vi "SwerveDriveLogic.vi"(8 "Joystick Axes":dbl[](array[numeric]), 9 "Speeds":dbl[](array[numeric]), 10 "AngleSetpoints":dbl[](array[numeric]), 11 "AngleEncoders":dbl[](array[numeric])) -> (2 "AngleMotorsReversed":bool[](array[boolean]), 3 "AngleMotorOutputs":dbl[](array[numeric]))   [LabVIEW 2018]
uses:
  <vilib>/addons/control/pid/pid.llb/PID (DBL).vi
  <vilib>/addons/control/pid/NI_PID_pid.lvlib
panel:
  out "Back right module":dbl(knob)
  out "Back left module":dbl(knob)
  out "Front left module":dbl(knob)
  out "Front right module":dbl(knob)
  in  "PID gains":T1={"proportional gain (Kc)"=0.02, "integral time (Ti, min)"=0.0, "derivative time (Td, min)"=0.0} {"derivative time (Td, min)" format="%.15f"; "integral time (Ti, min)" format="%.3f"; "proportional gain (Kc)" format="%.3f"}
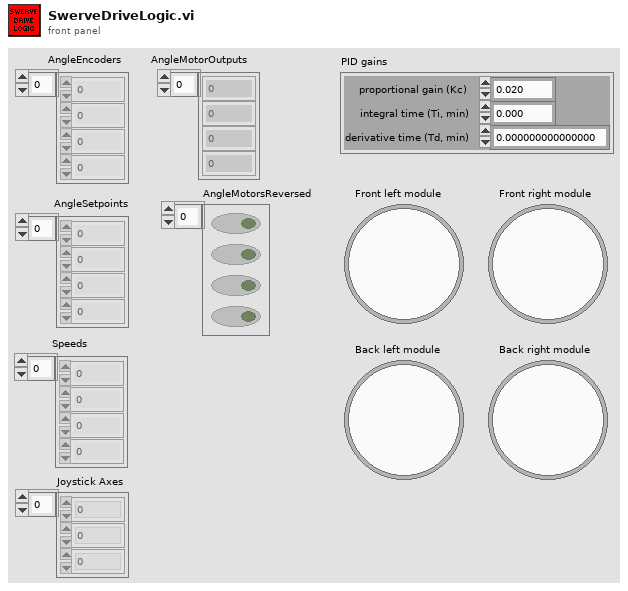
[diagram p1: front panel]
types:
  T1 = cluster{"proportional gain (Kc)":dbl, "integral time (Ti, min)":dbl, "derivative time (Td, min)":dbl}
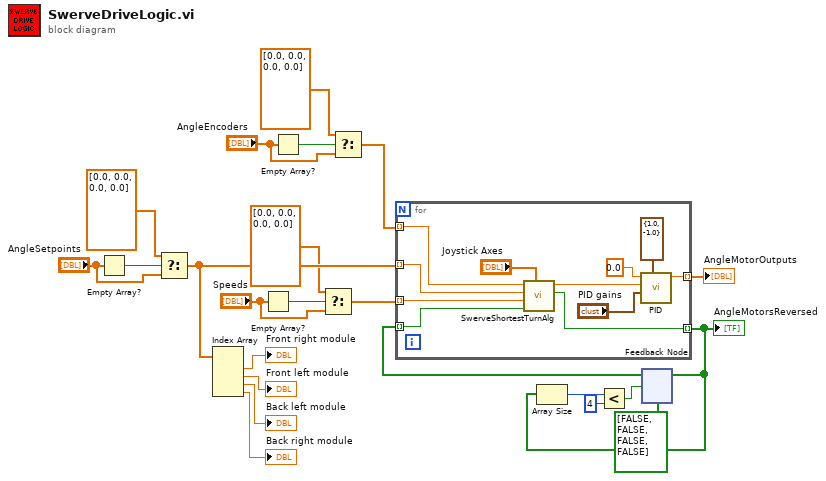
[diagram p0: block diagram]
diagram:
  n1 = Empty Array?(array="AngleSetpoints") -> (empty?=w15:bool)
  n2 = Select(t=dbl[] [0.0, 0.0, 0.0, 0.0] ("AngleSetpoints"), s=w15, f="AngleSetpoints") -> (s? t:f=w14:dbl[])
  n3 = Index Array(array=w14) -> (element #1=→"Front right module":dbl, element #2=→"Front left module":dbl, element #3=→"Back left module":dbl, element #4=→"Back right module":dbl)  [unwired: 4 in]
  n4 = Empty Array?(array="Speeds") -> (empty?=w12:bool)
  n5 = Empty Array?(array="AngleEncoders") -> (empty?=w18:bool)
  n6 = Select(t=dbl[] [0.0, 0.0, 0.0, 0.0] ("AngleSetpoints"), s=w12, f="Speeds") -> (s? t:f=w10:dbl[])
  n7 = Select(t=dbl[] [0.0, 0.0, 0.0, 0.0] ("AngleSetpoints"), s=w18, f="AngleEncoders") -> (s? t:f=w7:dbl[])
  n8 = feedback #1(bool[] [FALSE, FALSE, FALSE, FALSE]) -> (w3:bool[])
  n9 = for {
    tunnel: w3 -> [w29] mode=indexing
    tunnel: w14 -> [w31] mode=indexing
    tunnel: [w33] -> w23 mode=indexing
    tunnel: [w25] -> w2 mode=indexing
    tunnel: w7 -> [w28] mode=indexing
    tunnel: w10 -> [w27] mode=indexing
    n10 = call "SwerveShortestTurnAlg.vi"("Joystick Axes"="Joystick Axes", "SwerveMotorsFlipped?"=w29, "SwerveSpeed"=w27, "AngleSetpoint"=w31, "AngleEncoder"=w28) -> ("FlipSwerveMotors"=w25:bool, "PIDInput"=w26:dbl)  [unwired: 5 in]
    n11 = call-poly <vilib>:"PID.vi"("output range"=cluster{"output high":dbl, "output low":dbl} {"output high"=1.0, "output low"=-1.0}, "PID gains"="PID gains", "process variable"=w26, "setpoint"=0.0) -> ("output"=w33:dbl)  [unwired: 6 in, 1 out]
  }
  "AngleMotorsReversed" <- w2
  "AngleMotorOutputs" <- w23
  n12 = Array Size(array=w2) -> (size(s)=w4:i32)
  n13 = Less?(x=w4, y=4) -> (x < y?=w5:bool)
  n14 = feedback-in #1(w2, w5) -> ()
